vi "_Update Ion Path.vi"(0 "Value":dbl, 4 "Source Map":refnum<vi>, 5 "Current Cell":T1, 6 "Voltage OK":bool, 7 "ADC Ch#":u8=32, 8 "Lens Table":refnum<vi>, 9 "Ion Path":refnum<vi>) -> ()   [LabVIEW 2012]
uses:
  <vilib>/Utility/miscctls.llb/LVRowAndColumnTypeDef.ctl
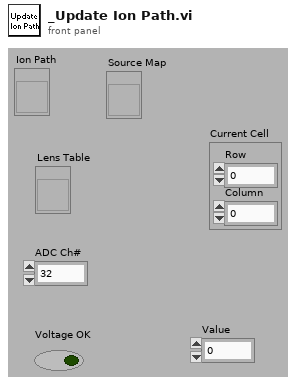
[diagram p1: front panel]
types:
  T1 = typedef "LVRowAndColumnTypeDef.ctl" = cluster{"Row":i32, "Column":i32}
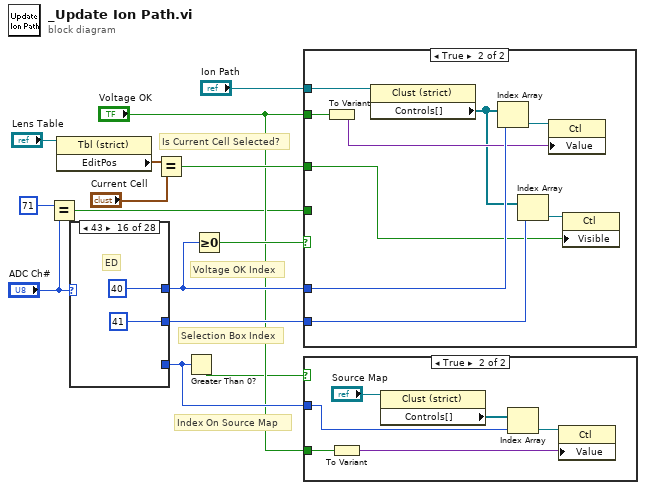
[diagram p0: block diagram]
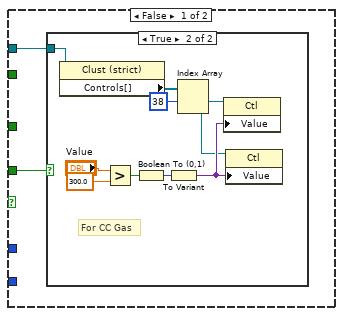
[diagram p3: hidden frame]
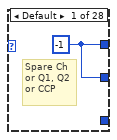
[diagram p5: hidden frame]
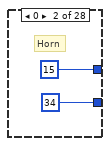
[diagram p6: hidden frame]
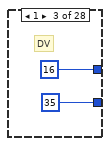
[diagram p7: hidden frame]
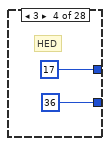
[diagram p8: hidden frame]
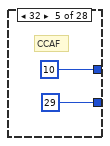
[diagram p9: hidden frame]
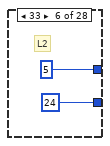
[diagram p10: hidden frame]
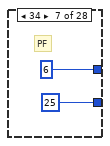
[diagram p11: hidden frame]
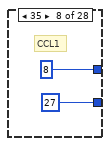
[diagram p12: hidden frame]
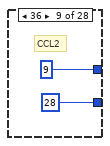
[diagram p13: hidden frame]
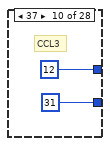
[diagram p14: hidden frame]
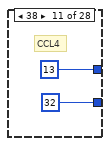
[diagram p15: hidden frame]
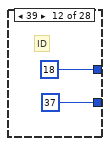
[diagram p16: hidden frame]
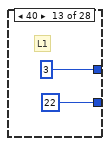
[diagram p17: hidden frame]
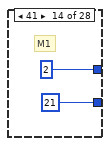
[diagram p18: hidden frame]
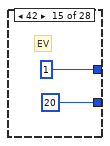
[diagram p19: hidden frame]
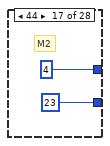
[diagram p20: hidden frame]
diagram:
  # "Index On Source Map"
  # "Selection Box Index"
  # "Voltage OK Index"
  # "Is Current Cell Selected?"
  n1 = Equal?(x=u8 71, y="ADC Ch#") -> (x = y?=w2:bool)
  n2 = property class="Tbl (strict)"(reference="Lens Table") -> ("EditPos"=w13:T1)  [unwired: 1 in, 2 out]
  n3 = case shown="43" "ADC Ch#" {
    tunnel: [w15 15 ("index") 16 ("index") 17 ("index") 10 ("index") 5 ("index") 6 ("index") 8 ("index") 9 ("index") 12 ("index") 13 ("index") 18 ("index") 3 ("index") 2 ("index") 1 ("index") 40 ("index") 4 ("index") 11 ("index") 0 ("index") -1 ("index") -1 ("index") -1 ("index") -1 ("index") -1 ("index") -1 ("index") -1 ("index") -1 ("index") -1 ("index")] -> w10
    tunnel: [w15 34 ("index") 35 ("index") 36 ("index") 29 ("index") 24 ("index") 25 ("index") 27 ("index") 28 ("index") 31 ("index") 32 ("index") 37 ("index") 22 ("index") 21 ("index") 20 ("index") 41 ("index") 23 ("index") 30 ("index") 19 ("index") _ _ _ _ _ _ _ _ _] -> w9
    tunnel: [_ _ _ _ _ _ _ _ _ _ _ _ _ _ _ _ _ _ 8 ("index") 2 ("index") 4 ("index") 11 ("index") 10 ("index") 6 ("index") 5 ("index") 9 ("index") 7 ("index") 3 ("index")] -> w8
    frame Default {
      w15 = -1 ("index")
      # "Spare Ch\nor Q1, Q2\nor CCP"
    }
    frame 0 {
      # "Horn"
    }
    frame 1 {
      # "DV"
    }
    frame 3 {
      # "HED"
    }
    frame 32 {
      # "CCAF"
    }
    frame 33 {
      # "L2"
    }
    frame 34 {
      # "PF"
    }
    frame 35 {
      # "CCL1"
    }
    frame 36 {
      # "CCL2"
    }
    frame 37 {
      # "CCL3"
    }
    frame 38 {
      # "CCL4"
    }
    frame 39 {
      # "ID"
    }
    frame 40 {
      # "L1"
    }
    frame 41 {
      # "M1"
    }
    frame 42 {
      # "EV"
    }
    frame 43 {
      # "ED"
    }
    frame 44 {
      # "M2"
    }
    frame 45 {
      # "CC"
    }
    frame 104 {
      # "CAP"
    }
    frame 106 {
      # "CD"
    }
    frame 64 {
      # "DG"
    }
    frame 65 {
      # "NG1"
    }
    frame 67 {
      # "HG1"
    }
    frame 66 {
      # "NG2"
    }
    frame 68 {
      # "HG2"
    }
    frame 70 {
      # "SX"
    }
    frame 107 {
      # "ESI 1"
    }
    frame 109 {
      # "ESI 2"
    }
  }
  n4 = Equal?(x=w13, y="Current Cell") -> (x = y?=w11:bool)
  n5 = Greater Than 0?(x=w8) -> (x > 0?=w5:bool)
  n6 = Greater Or Equal To 0?(x=w10) -> (x >= 0?=w7:bool)
  n7 = case shown="True" w7 {
    tunnel: w11 -> [_ w84]
    tunnel: "Voltage OK" -> [_ w89]
    tunnel: w10 -> [_ w91]
    tunnel: w9 -> [_ w86]
    tunnel: "Ion Path" -> [w71 w83]
    tunnel: w2 -> [w72 _]
    frame False {
      n8 = case shown="True" w72 {
        tunnel: w71 -> [_ w82]
        frame False {
        }
        frame True {
          # "For CC Gas"
          n9 = property class="Clust (strict)"(reference=w82) -> ("Controls[]"=w76:refnum<vi>[])  [unwired: 1 in, 2 out]
          n10 = Greater?(x="Value", y=300.0) -> (0:w75:bool)
          n11 = Boolean To (0,1)(Boolean=w75) -> (0, 1=w79:i16)
          n12 = To Variant(anything=w79) -> (Variant=w74:variant)
          n13 = Index Array(array=w76, index #1=38 ("index")) -> (element #1=w80:refnum<vi>, element #2=w73:refnum<vi>)  [unwired: 1 in]
          n14 = property class="Ctl"(reference=w80, "Value"=w74) -> ()  [unwired: 1 in, 2 out]
          n15 = property class="Ctl"(reference=w73, "Value"=w74) -> ()  [unwired: 1 in, 2 out]
        }
      }
    }
    frame True {
      n16 = To Variant(anything=w89) -> (Variant=w88:variant)
      n17 = property class="Clust (strict)"(reference=w83) -> ("Controls[]"=w87:refnum<vi>[])  [unwired: 1 in, 2 out]
      n18 = Index Array(array=w87, index=w91) -> (element=w90:refnum<vi>)
      n19 = Index Array(array=w87, index=w86) -> (element=w85:refnum<vi>)
      n20 = property class="Ctl"(reference=w90, "Value"=w88) -> ()  [unwired: 1 in, 2 out]
      n21 = property class="Ctl"(reference=w85, "Visible"=w84) -> ()  [unwired: 1 in, 2 out]
    }
  }
  n22 = case shown="True" w5 {
    tunnel: w8 -> [_ w94]
    tunnel: "Voltage OK" -> [_ w93]
    frame False {
    }
    frame True {
      n23 = To Variant(anything=w93) -> (Variant=w92:variant)
      n24 = property class="Clust (strict)"(reference="Source Map") -> ("Controls[]"=w96:refnum<vi>[])  [unwired: 1 in, 2 out]
      n25 = Index Array(array=w96, index=w94) -> (element=w97:refnum<vi>)
      n26 = property class="Ctl"(reference=w97, "Value"=w92) -> ()  [unwired: 1 in, 2 out]
    }
  }
